vi "Interpolate 1D Array Initialization VI.vi"(8 "error in (no error)":errorcluster, 10 "Custom XML":string, 11 "Device Item Ref in":T1 format="%.0x") -> (0 "error out":errorcluster, 3 "Device Item Ref out":T1 format="%.0x")   [LabVIEW 2011, in "Interpolate 1D Array Custom Device.lvlib"]
uses:
  Interpolate 1D Array Custom Device.lvlib
  <vilib>/NI Veristand/Custom Device API/Custom Device Item Ref.ctl
  <vilib>/NI Veristand/Custom Device API/Custom Device Channel Type.ctl
  <vilib>/NI Veristand/Custom Device API/Custom Device Channel.ctl
  Spreadsheet Info.ctl
  Interpolate Options.ctl
  Global Property Names.vi
  <vilib>/NI Veristand/Custom Device API/Set Item Property (Variant).vi
  <vilib>/NI Veristand/Custom Device API/Custom Device API.lvlib
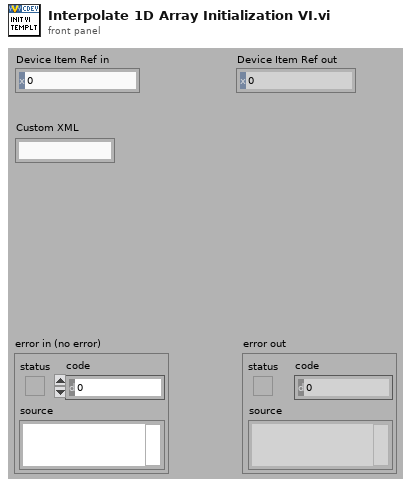
[diagram p1: front panel]
types:
  T1 = typedef "Custom Device API.lvlib/Custom Device Item Ref.ctl" = u64
  T2 = typedef "Custom Device API.lvlib/Custom Device Channel Type.ctl" = enum16{"Input", "Output"}
  T3 = typedef "Interpolate 1D Array Custom Device.lvlib/Spreadsheet Info.ctl" = cluster{"Delimiter":string, "Row Offset":dbl}
  T4 = typedef "Interpolate 1D Array Custom Device.lvlib/Interpolate Options.ctl" = cluster{"method":i32, "ntimes":i32, "X is monotonic":bool}
  T5 = typedef "Custom Device API.lvlib/Custom Device Channel.ctl" = cluster{"Type":T2, "Units":string, "Default Value":dbl, "Faultable":bool, "Scalable":bool}
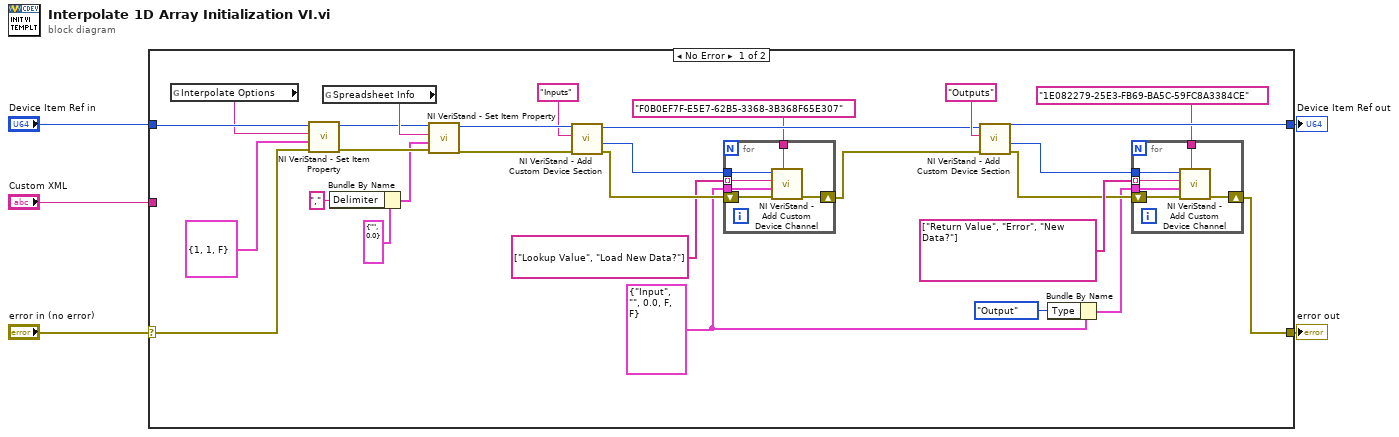
[diagram p0: block diagram]
diagram:
  n1 = case shown="No Error" "error in (no error)" {
    selector: "error in (no error)" -> [w31 w48]
    tunnel: [w8 w48] -> w5
    tunnel: [w9 w47] -> w3
    tunnel: "Device Item Ref in" -> [w34 w47]
    tunnel: "Custom XML" -> [_ _]
    frame No Error {
      w12 = T5 {"Type"=enum."Input", "Units"="", "Default Value"=0.0, "Faultable"=FALSE, "Scalable"=FALSE} ("Channel")
      n2 = global read "Global Property Names.vi" "Interpolate Options"() -> (w33:string)
      n3 = call-poly <vilib>:"NI VeriStand - Set Item Property.vi"("error in (no error)"=w31, "Value"=T4 {"method"=1, "ntimes"=1, "X is monotonic"=FALSE} ("Interpolate Options"), "Property Name"=w33, "Item Ref in"=w34) -> ("error out"=w28:errorcluster, "Item Ref out"=w29:T1)  [unwired: 5 in, 1 out]
      n4 = global read "Global Property Names.vi" "Spreadsheet Info"() -> (w30:string)
      n5 = Bundle By Name(cluster=T3 {"Delimiter"="", "Row Offset"=0.0} ("Spreadsheet Info"), "Delimiter"=",") -> (w23:T3)
      n6 = call-poly <vilib>:"NI VeriStand - Set Item Property.vi"("error in (no error)"=w28, "Value"=w23, "Property Name"=w30, "Item Ref in"=w29) -> ("error out"=w26:errorcluster, "Item Ref out"=w27:T1)  [unwired: 5 in, 1 out]
      n7 = call <vilib>:"NI VeriStand - Add Custom Device Section.vi"("error in (no error)"=w26, "Section Name"="Inputs", "Parent Ref in"=w27) -> ("error out"=w20:errorcluster, "Section Ptr"=w21:T1, "Parent Ref out"=w14:T1)  [unwired: 5 in, 1 out]
      n8 = for {
        tunnel: w21 -> [w46]
        shift-right: [w44] -> w13
        shift-left: w20 -> [w45]
        tunnel: string[] ["Lookup Value", "Load New Data?"] -> [w43] mode=indexing
        tunnel: w12 -> [w42]
        tunnel: "F0B0EF7F-E5E7-62B5-3368-3B368F65E307" -> [w41]
        n9 = call <vilib>:"NI VeriStand - Add Custom Device Channel.vi"("GUID (Default Channel)"=w41, "error in (no error)"=w45, "Channel"=w42, "Channel Name"=w43, "Parent Ref in"=w46) -> ("error out"=w44:errorcluster)  [unwired: 3 in, 3 out]
      }
      n10 = call <vilib>:"NI VeriStand - Add Custom Device Section.vi"("error in (no error)"=w13, "Section Name"="Outputs", "Parent Ref in"=w14) -> ("error out"=w17:errorcluster, "Section Ptr"=w16:T1, "Parent Ref out"=w9:T1)  [unwired: 5 in, 1 out]
      n11 = Bundle By Name(cluster=w12, "Type"=Custom_Device_Channel_Type."Output") -> (w10:T5)
      n12 = for {
        tunnel: w16 -> [w40]
        shift-right: [w38] -> w8
        shift-left: w17 -> [w39]
        tunnel: string[] ["Return Value", "Error", "New Data?"] -> [w37] mode=indexing
        tunnel: w10 -> [w36]
        tunnel: "1E082279-25E3-FB69-BA5C-59FC8A3384CE" -> [w35]
        n13 = call <vilib>:"NI VeriStand - Add Custom Device Channel.vi"("GUID (Default Channel)"=w35, "error in (no error)"=w39, "Channel"=w36, "Channel Name"=w37, "Parent Ref in"=w40) -> ("error out"=w38:errorcluster)  [unwired: 3 in, 3 out]
      }
    }
    frame Error {
    }
  }
  "error out" <- w5
  "Device Item Ref out" <- w3
